vi "RobStar.vi"() -> ()   [LabVIEW 2021]
panel:
  out "appended path":path
  out "string":string
  out "Array - String":string[](array[string])
  in  "python version":string="3.6"
  out "error out":errorcluster
  in  "error in (no error)":errorcluster
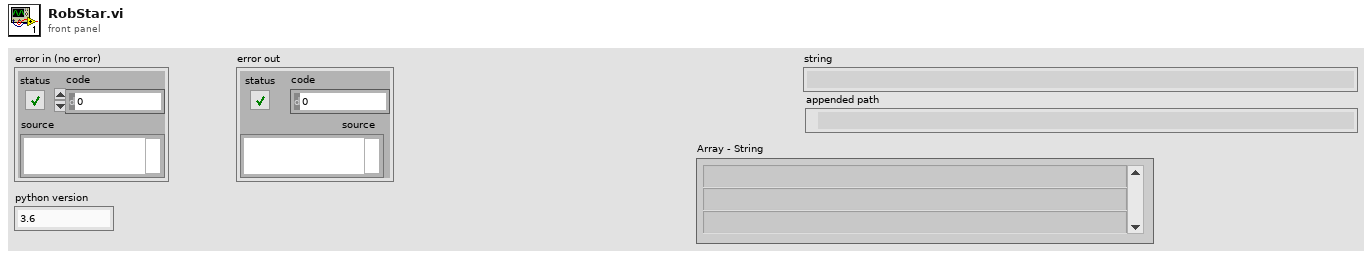
[diagram p1: front panel]
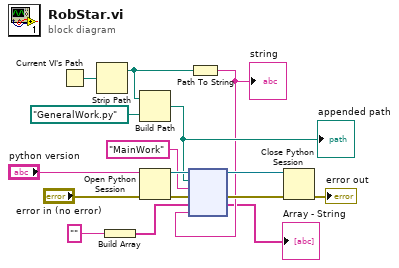
[diagram p0: block diagram]
diagram:
  n1 = Current VI's Path() -> (path=w7:path)
  n2 = Strip Path(path=w7) -> (stripped path=w5:path)  [unwired: 1 out]
  n3 = Build Array("") -> (w1:string[])
  n4 = Build Path(base path=w5, name or relative path=path "GeneralWork.py" ("python path")) -> (appended path=w9:path)
  "appended path" <- w9
  n5 = Open Python Session(python version="python version", 3:"error in (no error)") -> (session out=w14:refnum<k35>, error out=w13:errorcluster)  [unwired: 1 in]
  n6 = Path To String(path=w5) -> (string=w4:string)
  "string" <- w4
  n7 = node(w14, w9, "MainWork" ("function name in"), w13, w1, w4) -> (w16:refnum<k35>, w15:errorcluster, →"Array - String":string[])  [unwired: 1 in, 2 out]
  n8 = Close Python Session(session in=w16, error in=w15) -> (11:→"error out":errorcluster)
